vi "TeleOp Camera Servos.vi"   [LabVIEW 2020]
uses:
  <vilib>/Rock Robotics/WPI/Utilities/WPI_GetSetVariantRefNum.vi
types:
  T1 = typedef "WPI_JoystickDevRef.ctl" = cluster{"Device":T2}
  T2 = typedef "WPI_JoystickDeviceEnum.ctl" = enum16{"USB 0", "USB 1", "USB 2", "USB 3", "USB 4", "USB 5"}
  T3 = typedef "WPI_ServoDeviceRef.ctl" = cluster{"DeviceStatus":errorcluster, "PWM Channel":T4, "DeadBand":T5}
  T4 = typedef "FPGA_DIOPWMChannel.ctl" = enum8{"PWM 0", "PWM 1", "PWM 2", "PWM 3", "PWM 4", "PWM 5", "PWM 6", "PWM 7", "PWM 8", "PWM 9", "PWM MXP 0", "PWM MXP 1", "PWM MXP 2", "PWM MXP 3", "PWM MXP 4", "PWM MXP 5", "PWM MXP 6", "PWM MXP 7", "PWM MXP 8", "PWM MXP 9", "Invalid"}
  T5 = typedef "WPI_PWMDeadband.ctl" = cluster{"Name":string, "maxPositivePwm":i32, "minPositivePwm":i32, "centerPwm":i32, "maxNegativePwm":i32, "minNegativePwm":i32, "angularRange":u16}
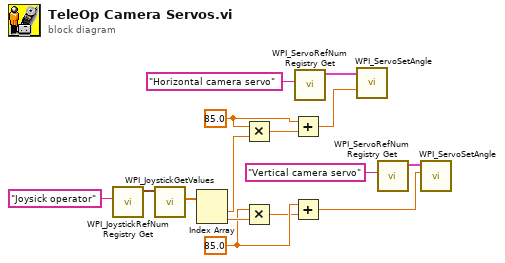
[diagram p0: block diagram]
diagram:
  w10 = 85.0 ("x")
  w7 = 85.0 ("x")
  n1 = call <vilib>:"WPI_JoystickRefNum Registry Get.vi"("refnum name"="Joysick operator") -> ("JoystickDevRef"=w2:T1)  [unwired: 9 in, 1 out]
  n2 = call <vilib>:"WPI_JoystickGetValues.vi"("JoystickDevRef"=w2) -> ("Axes"=w4:dbl[])  [unwired: 6 in, 4 out]
  n3 = Index Array(array=w4) -> (element #1=w5:dbl, element #2=w11:dbl)  [unwired: 2 in]
  n4 = Multiply(x=w7, y=w5) -> (x*y=w6:dbl)
  n5 = Multiply(x=w10, y=w11) -> (x*y=w9:dbl)
  n6 = Add(x=w7, y=w6) -> (x+y=w14:dbl)
  n7 = Add(x=w10, y=w9) -> (x+y=w13:dbl)
  n8 = call <vilib>:"WPI_ServoRefNum Registry Get.vi"("refnum name"="Horizontal camera servo") -> ("ServoDeviceRef"=w15:T3)  [unwired: 9 in, 1 out]
  n9 = call <vilib>:"WPI_ServoSetAngle.vi"("Angle"=w14, "ServoDeviceRef"=w15) -> ()  [unwired: 8 in, 2 out]
  n10 = call <vilib>:"WPI_ServoRefNum Registry Get.vi"("refnum name"="Vertical camera servo") -> ("ServoDeviceRef"=w12:T3)  [unwired: 9 in, 1 out]
  n11 = call <vilib>:"WPI_ServoSetAngle.vi"("Angle"=w13, "ServoDeviceRef"=w12) -> ()  [unwired: 8 in, 2 out]
